vi "Write IFD.vi"(0 "Byte Stream File in":refnum<file>, 1 "Additional Named Tags":cluster{"name":string, "Variant":variant}[](array[cluster]), 2 "Additional Tags":T2(array[cluster]), 3 "byte order (0:big-endian, network order)":T7(ring), 5 "IFD Offset Position":i64 format="%x", 9 "Offset":i64, 11 "error in":errorcluster, 12 "IFD Baseline":T6 {"SampleFormat" items=["UINT"=1, "INT"=2, "FP"=3, "VOID"=4, "COMPLEXINT"=5, "COMPLEXFP"=6]; "NewSubFileType" items=["FILETYPE_REDUCEDIMAGE"=1, "FILETYPE_PAGE"=2, "FILETYPE_MASK"=4]; "Compression" items=["COMPRESSION_NONE"=1, "COMPRESSION_CCITTRLE"=2, "COMPRESSION_CCITTFAX3"=3, "COMPRESSION_CCITTFAX4"=4, "COMPRESSION_LZW"=5, "COMPRESSION_OJPEG"=6, "COMPRESSION_JPEG"=7, "COMPRESSION_NEXT"=32766, "COMPRESSION_CCITTRLEW"=32771, "COMPRESSION_PACKBITS"=32773, "COMPRESSION_THUNDERSCAN"=32809, "COMPRESSION_IT8CTPAD"=32895, "COMPRESSION_IT8LW"=32896, "COMPRESSION_IT8MP"=32897, "COMPRESSION_IT8BL"=32898, "COMPRESSION_PIXARFILM"=32908, "COMPRESSION_PIXARLOG"=32909, "COMPRESSION_DEFLATE"=32946, "COMPRESSION_ADOBE_DEFLATE"=8, "COMPRESSION_DSC"=32947, "COMPRESSION_JBIG"=34661, "COMPRESSION_SGILOG"=34676, "COMPRESSION_SGILOG24"=34677, "COMPRESSION_JP2000"=34712]; "PhotometricInterpretation" items=["PHOTOMETRIC_MINISWHITE"=0, "PHOTOMETRIC_MINISBLACK"=1, "PHOTOMETRIC_RGB"=2, "PHOTOMETRIC_PALETTE"=3, "PHOTOMETRIC_MASK"=4, "PHOTOMETRIC_SEPARATED"=5, "PHOTOMETRIC_YCBCR"=6, "PHOTOMETRIC_CIELAB"=8, "PHOTOMETRIC_ICCLAB"=9, "PHOTOMETRIC_ITULAB"=10, "PHOTOMETRIC_LOGL"=32844, "PHOTOMETRIC_LOGLUV"=32845, "CFA"=32803, "LinearRaw"=34892, "DEPTH"=51177]; "ResolutionUnit" items=["RESUNIT_NONE"=1, "RESUNIT_INCH"=2, "RESUNIT_CENTIMETER"=3]}, 14 "Details":T3={"ImageDescription"="", "XResolution"=0.0, "YResolution"=0.0, "ResolutionUnit"=enum."Inch", "PhotometricInterpretation"=0, "Compression"=enum."None", "PageName"="", "DocumentName"=""} {"PhotometricInterpretation" items=["PHOTOMETRIC_MINISWHITE"=0, "PHOTOMETRIC_MINISBLACK"=1, "PHOTOMETRIC_RGB"=2, "PHOTOMETRIC_PALETTE"=3, "PHOTOMETRIC_MASK"=4, "PHOTOMETRIC_SEPARATED"=5, "PHOTOMETRIC_YCBCR"=6, "PHOTOMETRIC_CIELAB"=8, "PHOTOMETRIC_ICCLAB"=9, "PHOTOMETRIC_ITULAB"=10, "PHOTOMETRIC_LOGL"=32844, "PHOTOMETRIC_LOGLUV"=32845, "CFA"=32803, "LinearRaw"=34892, "DEPTH"=51177]}) -> (4 "refnum out":refnum<file>, 6 "Next IFD Offset Position":i64 format="%x", 10 "Next Offset":i64, 15 "error out":errorcluster)   [LabVIEW 2020, in "LV Tiff.lvlib"]
uses:
  LV Tiff.lvlib
  Baseline Tags 1.ctl
  Tiff Tag.ctl
  Tiff Tags.ctl
  Tiff Data Type.ctl
  Tiff Page Details.ctl
  de296096-4773-46d0-ada0-82523eb18cea.vi
  <vilib>/Comparison/Less/Less Functor/Less Functor.lvclass
  <vilib>/Utility/Data Type/NI_Data Type.lvlib
panel:
  out "Written Tags":T4[](array[typedef]) {"TagID" items=["NewSubfileType"=254, "ImageWidth"=256, "ImageLength"=257, "BitsPerSample"=258, "Compression"=259, "PhotometricInterpretation"=262, "StripOffsets"=273, "SamplesPerPixel"=277, "RowsPerStrip"=278, "StripByteCounts"=279, "XResolution"=282, "YResolution"=283, "ResolutionUnit"=296, "ColorMap"=320, "PlanarConfiguration"=284, "YCbCrCoefficients"=529, "YCbCrSubSampling"=530, "YCbCrPositioning"=531, "ReferenceBlackWhite"=532, "BadFaxLines"=326, "CleanFaxData"=327, "ConsecutiveBadFaxLines"=328, "SampleFormat"=339]}
  out "This IFD Position":u32
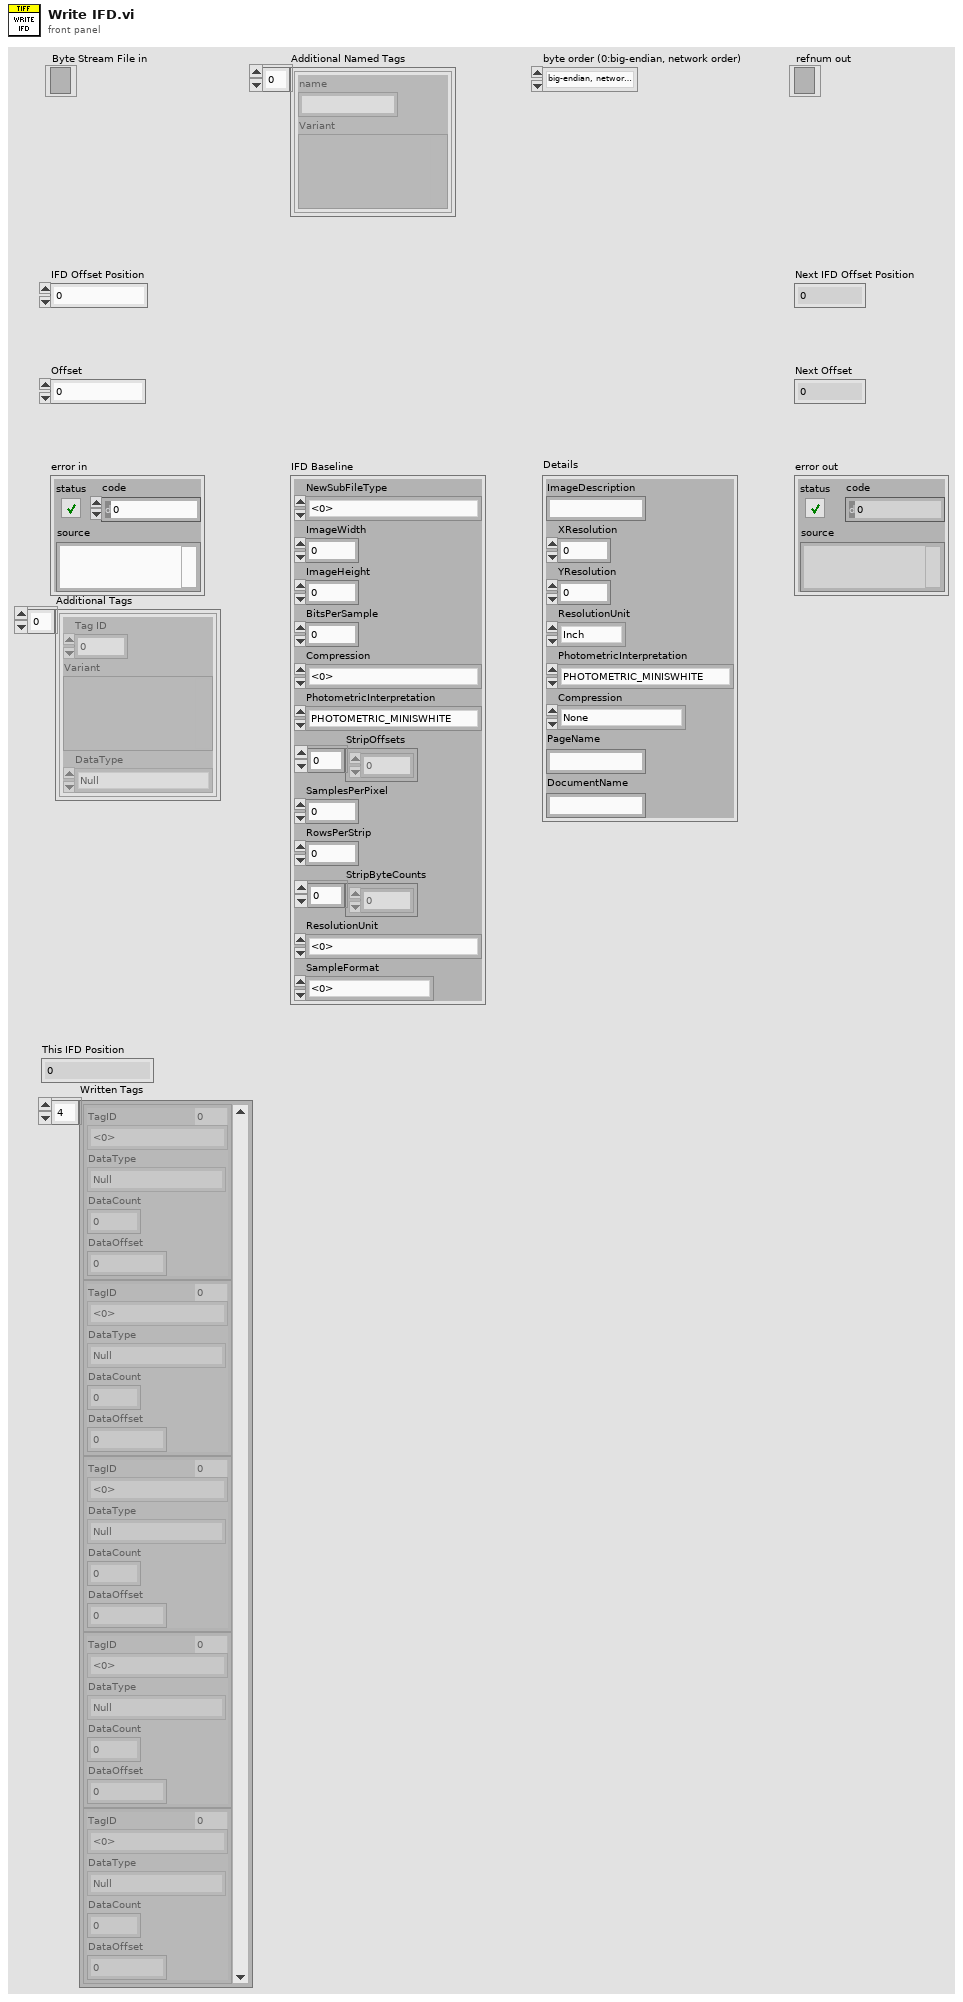
[diagram p1: front panel]
types:
  T1 = typedef "LV Tiff.lvlib/Tiff Data Type.ctl" = enum16{"Null", "BYTE", "ASCII", "SHORT", "LONG", "RATIONAL", "SBYTE", "UNDEFINE", "SSHORT", "SLONG", "SRATIONAL", "FLOAT", "DOUBLE"}
  T2 = cluster{"Tag ID":u32, "Variant":variant, "DataType":T1}[]
  T3 = typedef "LV Tiff.lvlib/Tiff Page Details.ctl" = cluster{"ImageDescription":string, "XResolution":dbl, "YResolution":dbl, "ResolutionUnit":enum16{"None", "Inch", "Centimeter"}, "PhotometricInterpretation":u16, "Compression":enum16{"None", "Deflate", "JPEG"}, "PageName":string, "DocumentName":string}
  T4 = typedef "LV Tiff.lvlib/Tiff Tag.ctl" = cluster{"TagID":T5, "DataType":T1, "DataCount":u32, "DataOffset":u32}
  T5 = typedef "LV Tiff.lvlib/Tiff Tags.ctl" = u16
  T6 = typedef "LV Tiff.lvlib/Baseline Tags 1.ctl" = cluster{"NewSubFileType":u32, "ImageWidth":u32, "ImageHeight":u32, "BitsPerSample":u16, "Compression":u16, "PhotometricInterpretation":u16, "StripOffsets":u32[], "SamplesPerPixel":u16, "RowsPerStrip":u32, "StripByteCounts":u32[], "ResolutionUnit":u16, "SampleFormat":u16}
  T7 = enum16{"big-endian, network order", "native, host order", "little-endian"}
  T8 = map{string, cluster{"Tag ID":u32, "Allowed Types":T1[]}}
  T9 = typedef "NI_Data Type.lvlib/Data Type.ctl" = enum8{"Invalid Type", "Void", "I8", "I16", "I32", "I64", "U8", "U16", "U32", "U64", "Single Float", "Double Float", "Extended Float", "Single Complex", "Double Complex", "Extended Complex", "Enum U8", "Enum U16", "Enum U32", "Enum U64", "Single Float With Unit", "Double Float With Unit", "Extended Float With Unit", "Single Complex with Unit", "Double Complex with Unit", "Extended Complex with Unit", "Boolean", "String", "Path", "Picture", "Tag", "Array", "Cluster", "Variant", "LV Variant", "Waveform", "Timestamp", "Digital Waveform", "Digital Data", "ExpressData", "Refnum", "External Data", "VI", "Poly VI", "LabVIEW Class Instance", "Fixed Point", "Set Collection", "Map Collection"}
  T10 = cluster{"Tag ID":u32, "Variant":variant, "type":T9, T1[]}
  T11 = cluster{"name":string, "Variant":variant, "type":T9}
  T12 = cluster{"name":string, "Variant":variant, "type":T9}[]
  T13 = cluster{"Tag ID":u32, "Variant":variant, "type":T9, "Allowed Types":T1[]}
  T14 = cluster{"Tag ID":u32, "Variant":variant, "type":T9, "Allowed Types":T1[]}[]
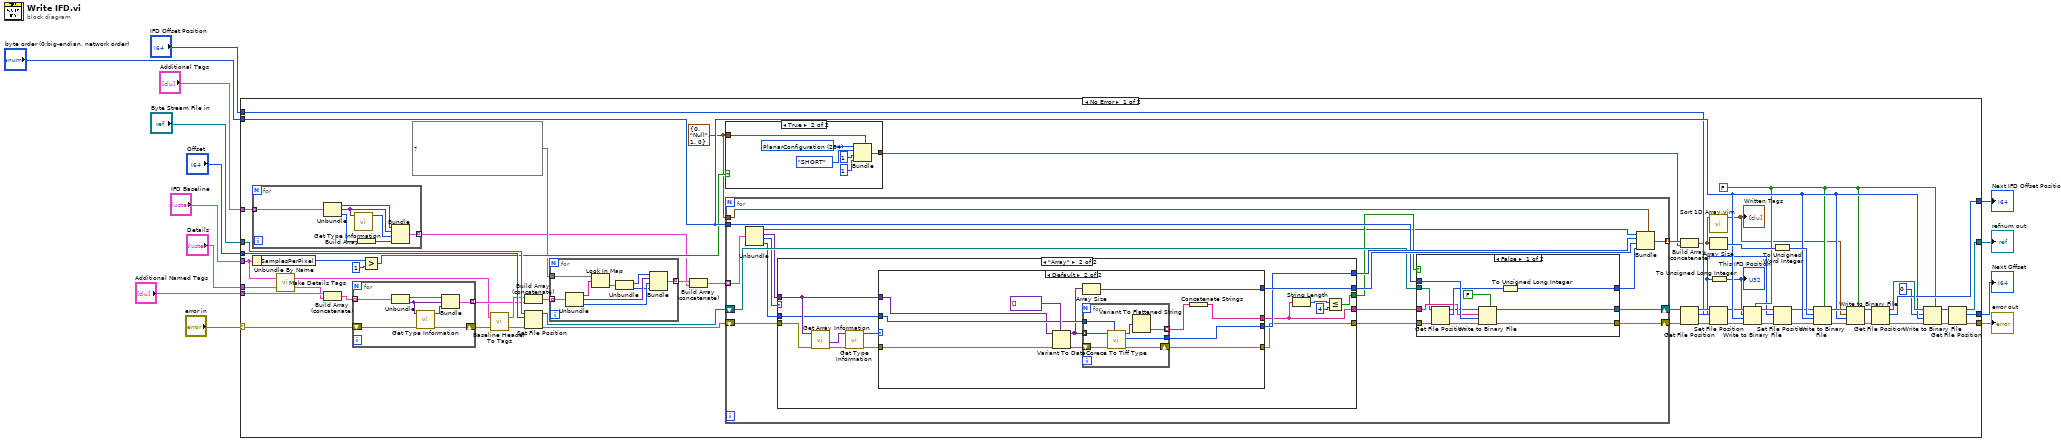
[diagram p0: block diagram]
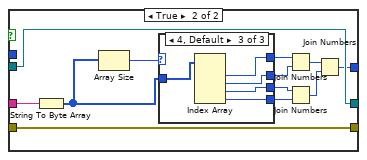
[diagram p3: hidden frame]
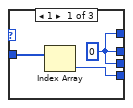
[diagram p4: hidden frame]
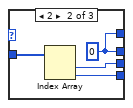
[diagram p5: hidden frame]
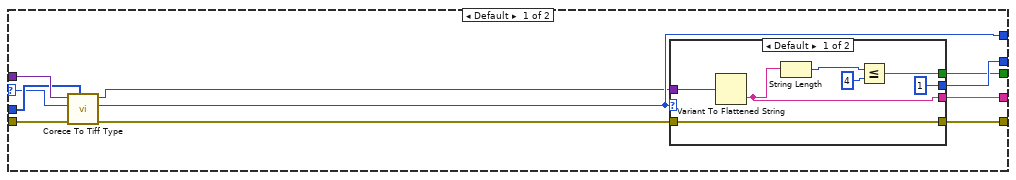
[diagram p6: hidden frame]
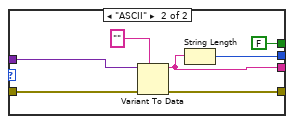
[diagram p7: hidden frame]
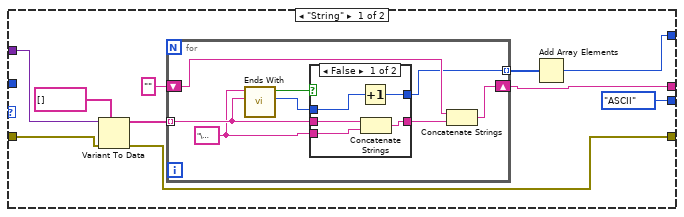
[diagram p8: hidden frame]
diagram:
  n1 = case shown="No Error" "error in" {
    selector: "error in" -> [w33 w238]
    tunnel: "Offset" -> [w72 _]
    tunnel: "Byte Stream File in" -> [w70 w237]
    tunnel: "IFD Baseline" -> [w22 _]
    tunnel: [w60 _] -> w10
    tunnel: [w56 w238] -> w8
    tunnel: [w54 w237] -> w7
    tunnel: [w53 _] -> w6
    tunnel: "byte order (0:big-endian, network order)" -> [w49 _]
    tunnel: "IFD Offset Position" -> [w44 _]
    tunnel: "Additional Named Tags" -> [w35 _]
    tunnel: "Details" -> [w23 _]
    tunnel: "Additional Tags" -> [w17 _]
    frame No Error {
      w48 = FALSE ("prepend array or string size? (T)")
      w25 = T4 {"TagID"=0, "DataType"=enum."Null", "DataCount"=1, "DataOffset"=0}
      n2 = for {
        tunnel: w17 -> [w79] mode=indexing
        tunnel: [w75] -> w15 mode=indexing
        n3 = Unbundle(w79) -> ("Tag ID"=w78:u32, "Variant"=w77:variant, "DataType"=w74:T1)
        n4 = call <vilib>:"Get Type Information.vi"("variant"=w77) -> ("type"=w76:T9)  [unwired: 6 in, 4 out]
        n5 = Build Array(w74) -> (w73:T1[])
        n6 = Bundle("Tag ID"=w78, "Variant"=w77, "type"=w76, w73) -> (w75:T10)  [unwired: 1 in]
      }
      n7 = Unbundle By Name(w22) -> ("SamplesPerPixel"=w28:u16)
      n8 = call "Make Details Tags.vi"("Details"=w23, "IFD Baseline"=w22) -> ("Tags"=w30:cluster{"name":string, "Variant":variant}[], "Modified IFD Baseline"=w21:T6)
      n9 = Build Array (concatenate)(w35, w30) -> (w31:cluster{"name":string, "Variant":variant}[])
      n10 = for {
        tunnel: w31 -> [w101] mode=indexing
        tunnel: [w97] -> w34 mode=indexing
        shift-right: [w95] -> w32
        shift-left: w33 -> [w96]
        n11 = Unbundle(w101) -> ("name"=w100:string, "Variant"=w99:variant)
        n12 = call <vilib>:"Get Type Information.vi"("error in (no error)"=w96, "variant"=w99) -> ("error out"=w95:errorcluster, "type"=w98:T9)  [unwired: 5 in, 3 out]
        n13 = Bundle("name"=w100, "Variant"=w99, "type"=w98) -> (w97:T11)  [unwired: 1 in]
      }
      n14 = Greater?(x=w28, y=u16 1) -> (0:w27:bool)
      n15 = call "Baseline Header To Tags.vi"("error in"=w32, "IFD Baseline"=w21) -> ("error out"=w37:errorcluster, "Tags"=w36:T12)
      n16 = Build Array (concatenate)(w36, w34) -> (w19:T12)
      n17 = Set File Position(offset (in bytes) (0)=w72, refnum=w70, error in=w37) -> (refnum out=w71:refnum<file>, error out=w58:errorcluster)  [unwired: 1 in]
      n18 = for {
        tunnel: T8 {"Artist"={"Tag ID"=315, "Allowed Types"=[enum."ASCII"]}, "BadFaxLines"={"Tag ID"=326, "Allowed Types"=[enum."SHORT", enum."LONG"]}, "BitsPerSample"={"Tag ID"=258, "Allowed Types"=[enum."SHORT"]}, "BlackIsZero"={"Tag ID"=1, "Allowed Types"=[]}, "CCITT 1D"={"Tag ID"=2, "Allowed Types"=[]}, "CCITT Group 3"={"Tag ID"=3, "Allowed Types"=[]}, "CCITT Group 4"={"Tag ID"=4, "Allowed Types"=[]}, "CIELab"={"Tag ID"=8, "Allowed Types"=[]}, "CMYK"={"Tag ID"=5, "Allowed Types"=[]}, "CellLength"={"Tag ID"=265, "Allowed Types"=[enum."SHORT"]}, "CellWidth"={"Tag ID"=264, "Allowed Types"=[enum."SHORT"]}, "CleanFaxData"={"Tag ID"=327, "Allowed Types"=[enum."SHORT"]}, "ColorMap"={"Tag ID"=320, "Allowed Types"=[enum."SHORT"]}, "ColorResponseCurve"={"Tag ID"=301, "Allowed Types"=[enum."SHORT"]}, "ColorResponseUnit"={"Tag ID"=300, "Allowed Types"=[enum."SHORT"]}, "Compression"={"Tag ID"=259, "Allowed Types"=[enum."SHORT"]}, "ConsecutiveBadFaxLines"={"Tag ID"=328, "Allowed Types"=[enum."LONG", enum."SHORT"]}, "Copyright"={"Tag ID"=33432, "Allowed Types"=[enum."ASCII"]}, "DateTime"={"Tag ID"=306, "Allowed Types"=[enum."ASCII"]}, "DocumentName"={"Tag ID"=269, "Allowed Types"=[enum."ASCII"]}, "DotRange"={"Tag ID"=336, "Allowed Types"=[enum."BYTE", enum."SHORT"]}, "ExtraSamples"={"Tag ID"=338, "Allowed Types"=[enum."BYTE"]}, "FillOrder"={"Tag ID"=266, "Allowed Types"=[enum."SHORT"]}, "FreeByteCounts"={"Tag ID"=289, "Allowed Types"=[enum."LONG"]}, "FreeOffsets"={"Tag ID"=288, "Allowed Types"=[enum."LONG"]}, "GrayResponseCurve"={"Tag ID"=291, "Allowed Types"=[enum."SHORT"]}, "GrayResponseUnit"={"Tag ID"=290, "Allowed Types"=[enum."SHORT"]}, "HalftoneHints"={"Tag ID"=321, "Allowed Types"=[enum."SHORT"]}, "HostComputer"={"Tag ID"=316, "Allowed Types"=[enum."ASCII"]}, "ImageDescription"={"Tag ID"=270, "Allowed Types"=[enum."ASCII"]}, "ImageHeight"={"Tag ID"=257, "Allowed Types"=[enum."SHORT", enum."LONG"]}, "ImageWidth"={"Tag ID"=256, "Allowed Types"=[enum."SHORT", enum."LONG"]}, "InkNames"={"Tag ID"=333, "Allowed Types"=[enum."ASCII"]}, "InkSet"={"Tag ID"=332, "Allowed Types"=[enum."SHORT"]}, "JPEG"={"Tag ID"=6, "Allowed Types"=[]}, "JPEGACTTables"={"Tag ID"=521, "Allowed Types"=[enum."LONG"]}, "JPEGDCTTables"={"Tag ID"=520, "Allowed Types"=[enum."LONG"]}, "JPEGInterchangeFormat"={"Tag ID"=513, "Allowed Types"=[enum."LONG"]}, "JPEGInterchangeFormatLength"={"Tag ID"=514, "Allowed Types"=[enum."LONG"]}, "JPEGLosslessPredictors"={"Tag ID"=517, "Allowed Types"=[enum."SHORT"]}, "JPEGPointTransforms"={"Tag ID"=518, "Allowed Types"=[enum."SHORT"]}, "JPEGProc"={"Tag ID"=512, "Allowed Types"=[enum."SHORT"]}, "JPEGQTables"={"Tag ID"=519, "Allowed Types"=[enum."LONG"]}, "JPEGRestartInterval"={"Tag ID"=515, "Allowed Types"=[enum."SHORT"]}, "LZW"={"Tag ID"=5, "Allowed Types"=[]}, "Make"={"Tag ID"=271, "Allowed Types"=[enum."ASCII"]}, "MaxSampleValue"={"Tag ID"=281, "Allowed Types"=[enum."SHORT"]}, "MinSampleValue"={"Tag ID"=280, "Allowed Types"=[enum."SHORT"]}, "Model"={"Tag ID"=272, "Allowed Types"=[enum."ASCII"]}, "NewSubFileType"={"Tag ID"=254, "Allowed Types"=[enum."LONG"]}, "NumberOfInks"={"Tag ID"=334, "Allowed Types"=[enum."SHORT"]}, "Orientation"={"Tag ID"=274, "Allowed Types"=[enum."SHORT"]}, "Packbits"={"Tag ID"=32773, "Allowed Types"=[]}, "PageName"={"Tag ID"=285, "Allowed Types"=[enum."ASCII"]}, "PageNumber"={"Tag ID"=297, "Allowed Types"=[enum."SHORT"]}, "PhotometricInterpretation"={"Tag ID"=262, "Allowed Types"=[enum."SHORT"]}, "PlanarConfiguration"={"Tag ID"=284, "Allowed Types"=[enum."SHORT"]}, "Predictor"={"Tag ID"=317, "Allowed Types"=[enum."SHORT"]}, "PrimaryChromaticities"={"Tag ID"=319, "Allowed Types"=[enum."RATIONAL"]}, "RGB"={"Tag ID"=2, "Allowed Types"=[]}, "RGB Palette"={"Tag ID"=3, "Allowed Types"=[]}, "ReferenceBlackWhite"={"Tag ID"=532, "Allowed Types"=[enum."LONG"]}, "ResolutionUnit"={"Tag ID"=296, "Allowed Types"=[enum."SHORT"]}, "RowsPerStrip"={"Tag ID"=278, "Allowed Types"=[enum."SHORT", enum."LONG"]}, "SMaxSampleValue"={"Tag ID"=341, "Allowed Types"=[enum."Null"]}, "SMinSampleValue"={"Tag ID"=340, "Allowed Types"=[enum."Null"]}, "SampleFormat"={"Tag ID"=339, "Allowed Types"=[enum."SHORT"]}, "SamplesPerPixel"={"Tag ID"=277, "Allowed Types"=[enum."SHORT"]}, "Software"={"Tag ID"=305, "Allowed Types"=[enum."ASCII"]}, "StripByteCounts"={"Tag ID"=279, "Allowed Types"=[enum."LONG", enum."SHORT"]}, "StripOffsets"={"Tag ID"=273, "Allowed Types"=[enum."SHORT", enum."LONG"]}, "SubFileType"={"Tag ID"=255, "Allowed Types"=[enum."SHORT"]}, "T4Options[2]"={"Tag ID"=292, "Allowed Types"=[enum."LONG"]}, "T6Options[3]"={"Tag ID"=293, "Allowed Types"=[enum."LONG"]}, "TargetPrinter"={"Tag ID"=337, "Allowed Types"=[enum."ASCII"]}, "Thresholding"={"Tag ID"=263, "Allowed Types"=[enum."SHORT"]}, "TileByteCounts"={"Tag ID"=325, "Allowed Types"=[enum."SHORT", enum."LONG"]}, "TileLength"={"Tag ID"=323, "Allowed Types"=[enum."SHORT", enum."LONG"]}, "TileOffsets"={"Tag ID"=324, "Allowed Types"=[enum."LONG"]}, "TileWidth"={"Tag ID"=322, "Allowed Types"=[enum."SHORT", enum."LONG"]}, "Tranparency Mask"={"Tag ID"=4, "Allowed Types"=[]}, "TransferFunction[4]"={"Tag ID"=301, "Allowed Types"=[enum."SHORT"]}, "TransferRange"={"Tag ID"=342, "Allowed Types"=[enum."SHORT"]}, "Uncompressed"={"Tag ID"=32771, "Allowed Types"=[]}, "WhiteIsZero"={"Tag ID"=0, "Allowed Types"=[]}, "WhitePoint"={"Tag ID"=318, "Allowed Types"=[enum."RATIONAL"]}, "XPosition"={"Tag ID"=286, "Allowed Types"=[enum."RATIONAL"]}, "XResolution"={"Tag ID"=282, "Allowed Types"=[enum."RATIONAL"]}, "YCbCr"={"Tag ID"=6, "Allowed Types"=[]}, "YCbCrCoefficients"={"Tag ID"=529, "Allowed Types"=[enum."RATIONAL"]}, "YCbCrPositioning"={"Tag ID"=531, "Allowed Types"=[enum."SHORT"]}, "YCbCrSubSampling"={"Tag ID"=530, "Allowed Types"=[enum."SHORT"]}, "YPosition"={"Tag ID"=287, "Allowed Types"=[enum."RATIONAL"]}, "YResolution"={"Tag ID"=283, "Allowed Types"=[enum."RATIONAL"]}} ("Map") -> [w88]
        tunnel: w19 -> [w87] mode=indexing
        tunnel: [w80] -> w18 mode=indexing
        n19 = Unbundle(w87) -> ("name"=w84:string, "Variant"=w83:variant, "type"=w82:T9)
        n20 = Look In Map(map=w88, key=w84) -> (value=w86:cluster{"Tag ID":u32, "Allowed Types":T1[]})  [unwired: 1 in, 1 out]
        n21 = Unbundle(w86) -> ("Tag ID"=w85:u32, "Allowed Types"=w81:T1[])
        n22 = Bundle("Tag ID"=w85, "Variant"=w83, "type"=w82, "Allowed Types"=w81) -> (w80:T13)  [unwired: 1 in]
      }
      n23 = Build Array (concatenate)(w18, w15) -> (w16:T14)
      n24 = case shown="True" w27 {
        tunnel: w25 -> [_ w94]
        tunnel: [_ w89] -> w24
        frame False {
        }
        frame True {
          w93 = T5 284 items=["NewSubfileType"=254, "ImageWidth"=256, "ImageLength"=257, "BitsPerSample"=258, "Compression"=259, "PhotometricInterpretation"=262, "StripOffsets"=273, "SamplesPerPixel"=277, "RowsPerStrip"=278, "StripByteCounts"=279, "XResolution"=282, "YResolution"=283, "ResolutionUnit"=296, "ColorMap"=320, "PlanarConfiguration"=284, "YCbCrCoefficients"=529, "YCbCrSubSampling"=530, "YCbCrPositioning"=531, "ReferenceBlackWhite"=532, "BadFaxLines"=326, "CleanFaxData"=327, "ConsecutiveBadFaxLines"=328, "SampleFormat"=339] ("Ring")
          n25 = Bundle(cluster=w94, "TagID"=w93, "DataType"=Tiff_Data_Type."SHORT", "DataCount"=u32 1, "DataOffset"=u32 1) -> (w89:T4)
        }
      }
      n26 = for {
        tunnel: w25 -> [w119]
        shift-right: [w116] -> w51
        shift-left: w71 -> [w115]
        tunnel: w49 -> [w113]
        tunnel: [w110] -> w69 mode=indexing
        shift-right: [w109] -> w59
        shift-left: w58 -> [w107]
        tunnel: w16 -> [w106] mode=indexing
        n27 = Unbundle(w106) -> ("Tag ID"=w103:u32, "Variant"=w104:variant, "type"=w105:T9, "Allowed Types"=w102:T1[])
        n28 = case shown="\"Array\"" w105 {
          selector: w105 -> [w155 _]
          tunnel: w104 -> [w165 w189]
          tunnel: [w161 w193] -> w118
          tunnel: [w162 w190] -> w117
          tunnel: [w156 w183] -> w111
          tunnel: [w158 w180] -> w112
          tunnel: w107 -> [w164 w188]
          tunnel: [w159 w185] -> w108
          tunnel: w102 -> [w163 w184]
          frame Default {
            n29 = call "Corece To Tiff Type.vi"("Allowed Types"=w163, "error in (no error)"=w164, "Variant Data type (optional)"=w155, "Variant"=w165) -> ("error out"=w160:errorcluster, "Actual Type"=w162:T1, "Coerced Variant"=w157:variant)  [unwired: 5 in]
            n30 = case shown="Default" w162 {
              tunnel: [u32 1 ("Size") w174] -> w161
              tunnel: w160 -> [w171 w179]
              tunnel: [w171 w178] -> w159
              tunnel: [w169 FALSE] -> w158
              tunnel: w157 -> [w167 w177]
              tunnel: [w166 w175] -> w156
              frame Default {
                n31 = Variant To Flattened String(Variant=w167) -> (data string=w166:string)  [unwired: 1 out]
                n32 = String Length(string=w166) -> (length=w168:i32)
                n33 = Less Or Equal?(x=w168, y=4) -> (x <= y?=w169:bool)
              }
              frame "ASCII" {
                n34 = Variant To Data(error in=w179, type="", Variant=w177) -> (data=w175:string, error out=w178:errorcluster)
                n35 = String Length(string=w175) -> (length=w174:i32)
              }
            }
          }
          frame "Array" {
            n36 = call <vilib>:"Get Array Information.vi"("error in (no error)"=w188, "variant"=w189) -> ("error out"=w187:errorcluster, "array element data type"=w192:variant)  [unwired: 6 in, 2 out]
            n37 = call <vilib>:"Get Type Information.vi"("error in (no error)"=w187, "variant"=w192) -> ("error out"=w186:errorcluster, "type"=w191:T9)  [unwired: 5 in, 3 out]
            n38 = case shown="Default" w191 {
              tunnel: [w198 w221] -> w193
              tunnel: [w196 w220] -> w183
              tunnel: [Tiff_Data_Type."ASCII" ("DataType") w224] -> w190
              tunnel: w189 -> [w203 w223]
              tunnel: w186 -> [w195 w229]
              tunnel: [w194 w226] -> w185
              tunnel: w184 -> [_ w225]
              frame "String" {
                n39 = Variant To Data(error in=w195, type=string[] [], Variant=w203) -> (data=w201:string[], error out=w194:errorcluster)
                n40 = for {
                  tunnel: w201 -> [w210] mode=indexing
                  shift-right: [w207] -> w196
                  shift-left: "" -> [w208]
                  tunnel: [w205] -> w199 mode=indexing
                  w209 = "\u0000" ("Suffix")
                  n41 = call "Ends With.vi"("String"=w210, "Suffix"=w209) -> ("String length"=w204:i32, "Ended with"=w211:bool)  [unwired: 8 in]
                  n42 = case shown="False" w211 {
                    tunnel: [w215 w218] -> w206
                    tunnel: w210 -> [w216 w218]
                    tunnel: w209 -> [w214 _]
                    tunnel: [w212 w217] -> w205
                    tunnel: w204 -> [w213 w217]
                    frame False {
                      n43 = Increment(x=w213) -> (x+1=w212:i32)
                      n44 = Concatenate Strings(w216, w214) -> (w215:string)
                    }
                    frame True {
                    }
                  }
                  n45 = Concatenate Strings(w208, w206) -> (w207:string)
                }
                n46 = Add Array Elements(numeric array=w199) -> (sum=w198:i32)
              }
              frame Default {
                n47 = Variant To Data(error in=w229, type=variant[] [], Variant=w223) -> (data=w222:variant[], error out=w227:errorcluster)
                n48 = Array Size(array=w222) -> (size(s)=w221:i32)
                n49 = for {
                  tunnel: w222 -> [w234] mode=indexing
                  shift-right: [w235] -> w226
                  shift-left: w227 -> [w236]
                  tunnel: w225 -> [w233]
                  tunnel: [w232] -> w224
                  tunnel: [w230] -> w219 mode=indexing
                  n50 = call "Corece To Tiff Type.vi"("Allowed Types"=w233, "error in (no error)"=w236, "Variant"=w234) -> ("error out"=w235:errorcluster, "Actual Type"=w232:T1, "Coerced Variant"=w231:variant)  [unwired: 6 in]
                  n51 = Variant To Flattened String(Variant=w231) -> (data string=w230:string)  [unwired: 1 out]
                }
                n52 = Concatenate Strings(w219) -> (w220:string)
              }
            }
            n53 = String Length(string=w183) -> (length=w182:i32)
            n54 = Less Or Equal?(x=w182, y=4) -> (x <= y?=w180:bool)
          }
        }
        n55 = case shown="False" w112 {
          tunnel: [w121 w142] -> w116
          tunnel: w115 -> [w126 w142]
          tunnel: w111 -> [w127 w141]
          tunnel: [w120 w134] -> w114
          tunnel: w113 -> [w130 _]
          tunnel: [w122 w133] -> w109
          tunnel: w108 -> [w124 w133]
          frame False {
            n56 = Get File Position(4:w124, 7:w126) -> (0:w123:errorcluster, 2:w128:i64, 3:w125:refnum<file>)
            n57 = Write to Binary File(file (use dialog)=w125, data=w127, error in=w123, 5:FALSE ("prepend array or string size? (T)"), 9:w130) -> (refnum out=w121:refnum<file>, error out=w122:errorcluster)  [unwired: 1 in, 1 out]
            n58 = To Unsigned Long Integer(number=w128) -> (unsigned 32bit integer=w120:u32)
          }
          frame True {
            n59 = String To Byte Array(string=w141) -> (unsigned byte array=w132:u8[])
            n60 = Array Size(array=w132) -> (size(s)=w131:i32)
            n61 = case shown="4, Default" w131 {
              tunnel: [w143 w146 w154] -> w140
              tunnel: [w143 w146 w153] -> w139
              tunnel: [w143 w148 w152] -> w138
              tunnel: [w144 w147 w151] -> w137
              tunnel: w132 -> [w145 w149 w150]
              frame 1 {
                w143 = u8 0
                n62 = Index Array(array=w145) -> (element=w144:u8)  [unwired: 1 in]
              }
              frame 2 {
                w146 = u8 0
                n63 = Index Array(array=w149) -> (element #1=w148:u8, element #2=w147:u8)  [unwired: 2 in]
              }
              frame 4, Default {
                n64 = Index Array(array=w150) -> (element #1=w154:u8, element #2=w153:u8, element #3=w152:u8, element #4=w151:u8)  [unwired: 4 in]
              }
            }
            n65 = Join Numbers(hi=w140, lo=w139) -> ((hi.lo)=w136:u16)
            n66 = Join Numbers(hi=w138, lo=w137) -> ((hi.lo)=w135:u16)
            n67 = Join Numbers(hi=w136, lo=w135) -> ((hi.lo)=w134:u32)
          }
        }
        n68 = Bundle(cluster=w119, "TagID"=w103, "DataType"=w117, "DataCount"=w118, "DataOffset"=w114) -> (w110:T4)
      }
      n69 = Build Array (concatenate)(w69, w24) -> (w29:T4[])
      n70 = Get File Position(4:w59, 7:w51) -> (0:w52:errorcluster, 2:w40:i64, 3:w46:refnum<file>)
      n71 = call "Sort 1D Array.vim"("unsorted array"=w29) -> ("sorted array"=w38:T4[])  [unwired: 10 in]
      "Written Tags" <- w38
      n72 = Array Size(array=w29) -> (size(s)=w68:i32)
      n73 = To Unsigned Long Integer(number=w40) -> (unsigned 32bit integer=w39:u32)
      "This IFD Position" <- w39
      n74 = Set File Position(offset (in bytes) (0)=w44, refnum=w46, error in=w52) -> (refnum out=w45:refnum<file>, error out=w47:errorcluster)  [unwired: 1 in]
      n75 = Write to Binary File(file (use dialog)=w45, data=w39, error in=w47, 5:w48, 9:w49) -> (refnum out=w42:refnum<file>, error out=w50:errorcluster)  [unwired: 1 in, 1 out]
      n76 = To Unsigned Word Integer(number=w68) -> (unsigned 16bit integer=w67:u16)
      n77 = Set File Position(offset (in bytes) (0)=w40, refnum=w42, error in=w50) -> (refnum out=w41:refnum<file>, error out=w43:errorcluster)  [unwired: 1 in]
      n78 = Write to Binary File(file (use dialog)=w41, data=w67, error in=w43, 5:w48, 9:w49) -> (refnum out=w65:refnum<file>, error out=w66:errorcluster)  [unwired: 1 in, 1 out]
      n79 = Write to Binary File(file (use dialog)=w65, data=w38, error in=w66, 5:w48, 9:w49) -> (refnum out=w62:refnum<file>, error out=w64:errorcluster)  [unwired: 1 in, 1 out]
      n80 = Get File Position(4:w64, 7:w62) -> (0:w63:errorcluster, 2:w60:i64, 3:w61:refnum<file>)
      n81 = Write to Binary File(file (use dialog)=w61, data=u32 0, error in=w63, 5:w48, 9:w49) -> (refnum out=w55:refnum<file>, error out=w57:errorcluster)  [unwired: 1 in, 1 out]
      n82 = Get File Position(4:w57, 7:w55) -> (0:w56:errorcluster, 2:w53:i64, 3:w54:refnum<file>)
    }
    frame Error {
    }
  }
  "Next IFD Offset Position" <- w10
  "refnum out" <- w7
  "error out" <- w8
  "Next Offset" <- w6
